vi "Display status.vi"(7 "action":enum16{"Init", "Get", "Set"}(ring)=enum."Set", 8 "error in":errorcluster, 11 "display status in":bool) -> (0 "error out":errorcluster, 3 "display status out":bool)   [LabVIEW 2018]
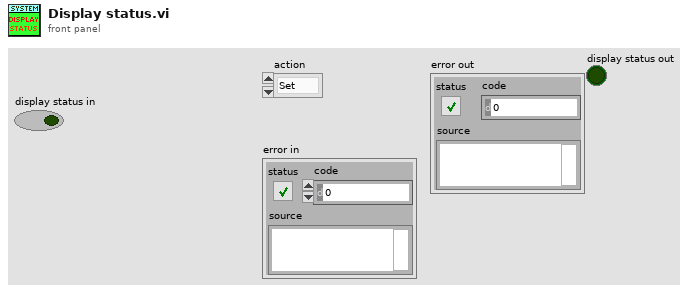
[diagram p1: front panel]
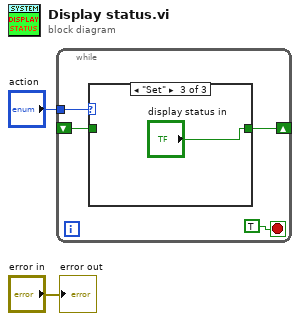
[diagram p0: block diagram]
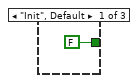
[diagram p2: hidden frame]
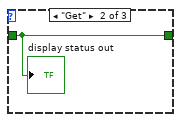
[diagram p3: hidden frame]
diagram:
  n1 = while {
    tunnel: "action" -> [w5]
    shift-right: [w3] -> _
    shift-left: _ -> [w4]
    stop <- TRUE stop-if-true
    n2 = case shown="\"Set\"" w5 {
      tunnel: w4 -> [_ w8 _]
      tunnel: [FALSE w8 "display status in"] -> w3
      frame "Init", Default {
      }
      frame "Get" {
        "display status out" <- w8
      }
      frame "Set" {
      }
    }
  }
  "error out" <- "error in"
